vi "6700C Wrapper.vi"(6 "Measurement Type":i32(ring)=1 items=["Current", "Voltage", "Power"], 7 "States":T2, 8 "error in":errorcluster, 9 "Enable Output":bool, 10 "Setting":T1={"Max Volt"=10.0, "Voltage Set"=0.01, "Current Lim"=0.5, "Source Type"=enum."Current", "Current Set"=0.01, "Max Current"=10.0, "Voltage Lim"=0.5}, 11 "Alias":string="PS1") -> (0 "error out":errorcluster, 1 "Error Message":string, 2 "Error":i32, 3 "Measurement":dbl=nan)   [LabVIEW 2021]
doc: "This is a wrapper to support Keysight N6700C."
uses:
  Controls/PS States.ctl
  Load INI/Controls/PowerSupply_Data.ctl
  <instrlib>/Agilent N6700 Series/Agilent N6700 Series.lvlib
panel:
  # "This wrapper has only been tested with N6773A and\nN6744B PS Modules (loaded in N6700C mainframe\nall other models are disabled unless tested and added to list"
  # "Voltage Src"
  # "Current Src"
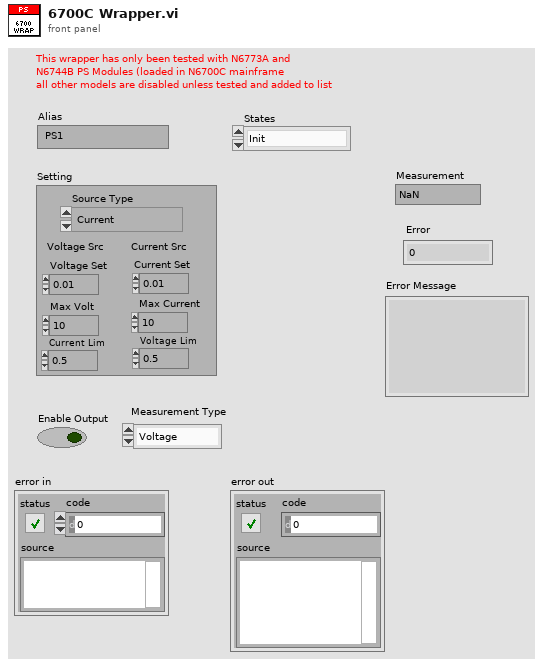
[diagram p1: front panel]
types:
  T1 = cluster{"Max Volt":dbl, "Voltage Set":dbl, "Current Lim":dbl, "Source Type":enum16{"Voltage", "Current"}, "Current Set":dbl, "Max Current":dbl, "Voltage Lim":dbl}
  T2 = typedef "PS States.ctl" = enum16{"Init", "Config", "Enable Output", "Measure", "Close"}
  T3 = cluster{"Channel Name":string, "VISA resource name":refnum<visa-resource-name>}
  T4 = typedef "PowerSupply_Data.ctl" = cluster{"Alias":string, "Device":string, "Channel name":string}
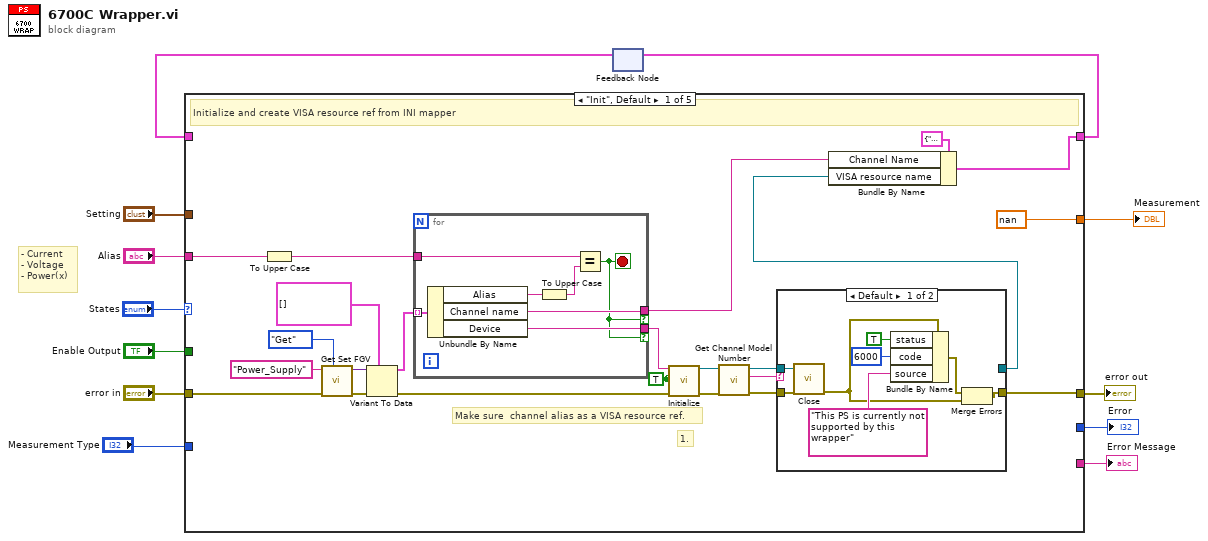
[diagram p0: block diagram]
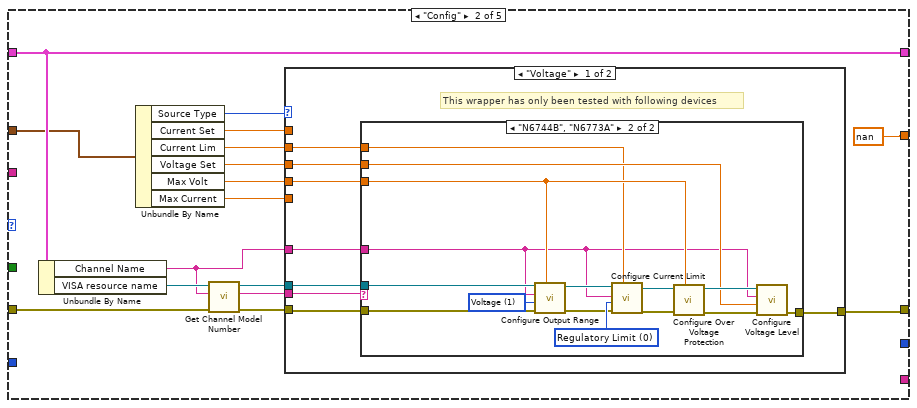
[diagram p3: hidden frame]
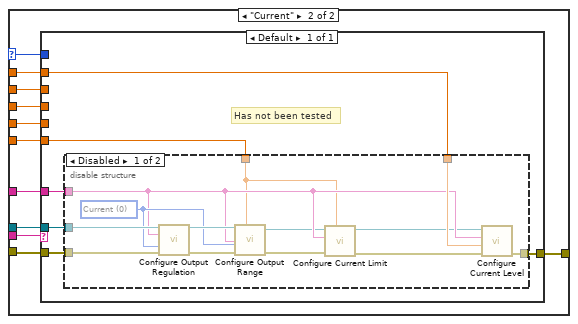
[diagram p5: hidden frame]
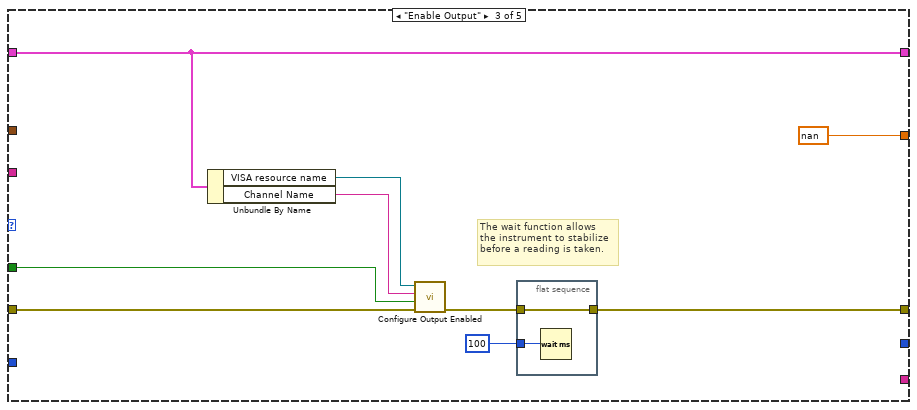
[diagram p7: hidden frame]
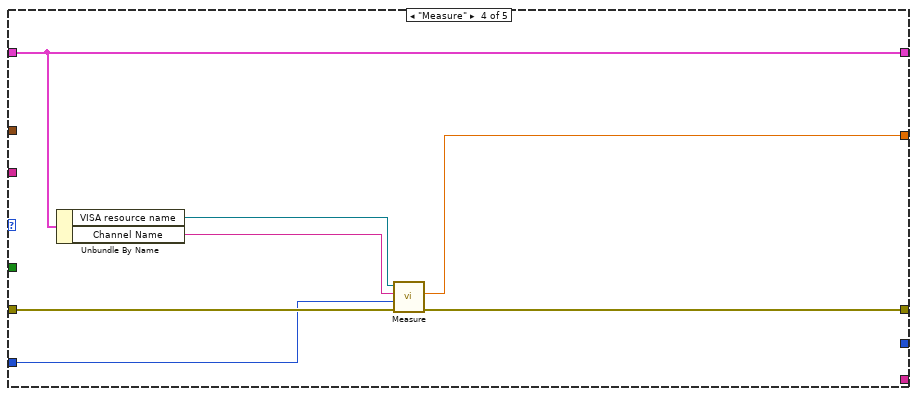
[diagram p8: hidden frame]
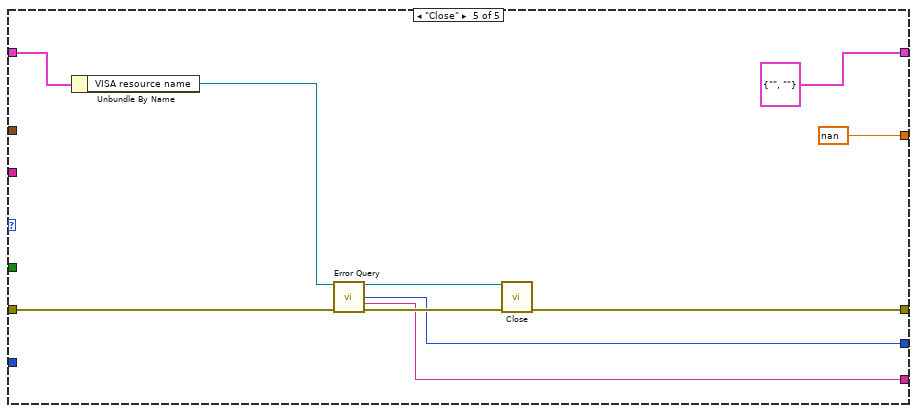
[diagram p9: hidden frame]
diagram:
  # "- Current\n- Voltage\n- Power(x)"
  n1 = feedback #1() -> (w8:T3)  [unwired: 1 in]
  n2 = case shown="\"Init\", Default" "States" {
    tunnel: "error in" -> [w33 w66 w132 w138 w148]
    tunnel: [w15 w61 w126 w140 w144] -> w10
    tunnel: [w34 w68 w131 w139 T3 {"Channel Name"="", "VISA resource name"=""}] -> w9
    tunnel: w8 -> [_ w68 w131 w139 w151]
    tunnel: [nan nan nan w141 nan] -> w4
    tunnel: "Enable Output" -> [_ _ w129 _ _]
    tunnel: "Setting" -> [_ w67 _ _ _]
    tunnel: "Alias" -> [w27 _ _ _ _]
    tunnel: [_ _ _ _ w143] -> w3
    tunnel: [_ _ _ _ w142] -> w2
    tunnel: "Measurement Type" -> [_ _ _ w135 _]
    frame "Init", Default {
      w23 = TRUE ("Reset? (T: Yes)")
      # "1."
      # "Make sure  channel alias as a VISA resource ref."
      # "Initialize and create VISA resource ref from INI mapper"
      n3 = To Upper Case(1:w27) -> (0:w26:string)
      n4 = call "Get Set FGV.vi"("Method (Get)"=enum16{"Get", "Set"}."Get", "error in"=w33, "Name"="Power_Supply") -> ("error out"=w31:errorcluster, "Data out"=w30:variant)  [unwired: 7 in]
      n5 = Variant To Data(error in=w31, type=T4[] [], Variant=w30) -> (data=w28:T4[], error out=w20:errorcluster)
      n6 = for {
        tunnel: w28 -> [w52] mode=indexing
        tunnel: w26 -> [w51]
        tunnel: [w48] -> w25 if=w46
        tunnel: [w47] -> w24 if=w46
        stop <- w46 stop-if-true
        n7 = Unbundle By Name(w52) -> ("Alias"=w49:string, "Channel name"=w47:string, "Device"=w48:string)
        n8 = To Upper Case(1:w49) -> (0:w50:string)
        n9 = Equal?(x=w51, y=w50) -> (x = y?=w46:bool)
      }
      n10 = call <instrlib>:"Initialize.vi"("VISA resource name"=w25, "ID Query? (T: Yes)"=w23, "Reset? (T: Yes)"=w23, "error in (no error)"=w20) -> ("VISA resource name out"=w18:refnum<visa-resource-name>, "error out"=w19:errorcluster)  [unwired: 10 in]
      n11 = call <instrlib>:"Get Channel Model Number.vi"("error in (no error)"=w19, "VISA resource name"=w18) -> ("error out"=w16:errorcluster, "Model Number"=w17:string, "VISA resource name out"=w14:refnum<visa-resource-name>)  [unwired: 7 in]
      n12 = case shown="Default" w17 {
        tunnel: w16 -> [w43 w45]
        tunnel: [w37 w45] -> w15
        tunnel: w14 -> [w42 w44]
        tunnel: [_ w44] -> w13
        frame Default {
          n13 = call <instrlib>:"Close.vi"("VISA resource name"=w42, "error in (no error)"=w43) -> ("error out"=w36:errorcluster)  [unwired: 13 in]
          n14 = Bundle By Name(cluster=w36, "status"=TRUE, "code"=6000, "source"="This PS is currently not supported by this wrapper") -> (w38:errorcluster)
          n15 = Merge Errors(w38, w36) -> (w37:errorcluster)
        }
        frame "N6744B", "N6773A" {
        }
      }
      n16 = Bundle By Name(cluster=T3 {"Channel Name"="", "VISA resource name"=""}, "Channel Name"=w24, "VISA resource name"=w13) -> (w34:T3)
    }
    frame "Config" {
      n17 = Unbundle By Name(w68) -> ("Channel Name"=w53:string, "VISA resource name"=w64:refnum<visa-resource-name>)
      n18 = Unbundle By Name(w67) -> ("Source Type"=w55:enum16{"Voltage", "Current"}, "Current Set"=w56:dbl, "Current Lim"=w60:dbl, "Voltage Set"=w58:dbl, "Max Volt"=w59:dbl, "Max Current"=w54:dbl)
      n19 = call <instrlib>:"Get Channel Model Number.vi"("error in (no error)"=w66, "Channel Name (1)"=w53, "VISA resource name"=w64) -> ("error out"=w65:errorcluster, "Model Number"=w57:string, "VISA resource name out"=w63:refnum<visa-resource-name>)  [unwired: 6 in]
      n20 = case shown="\"Voltage\"" w55 {
        selector: w55 -> [_ w94]
        tunnel: w53 -> [w70 w98]
        tunnel: w65 -> [w71 w102]
        tunnel: w63 -> [w72 w103]
        tunnel: [w75 w97] -> w61
        tunnel: w60 -> [w73 w101]
        tunnel: w59 -> [w74 w100]
        tunnel: w58 -> [w76 w99]
        tunnel: w57 -> [w69 w96]
        tunnel: w56 -> [_ w95]
        tunnel: w54 -> [_ w93]
        frame "Voltage" {
          # "This wrapper has only been tested with following devices"
          n21 = case shown="\"N6744B\", \"N6773A\"" w69 {
            tunnel: w76 -> [_ w86]
            tunnel: [w77 w84] -> w75
            tunnel: w74 -> [_ w83]
            tunnel: w73 -> [_ w82]
            tunnel: w72 -> [_ w81]
            tunnel: w71 -> [w77 w80]
            tunnel: w70 -> [_ w79]
            frame Default {
            }
            frame "N6744B", "N6773A" {
              w78 = 1 items=["Voltage"=1, "Current"=0] ("Range Type (1: Voltage)")
              w92 = 0 items=["Regulatory Limit", "Trip Limit"] ("Behavior (0: Regulatory Limit)")
              n22 = call <instrlib>:"Configure Output Range.vi"("Range (0.0)"=w83, "error in (no error)"=w80, "Range Type (1: Voltage)"=w78, "Channel Name (1)"=w79, "VISA resource name"=w81) -> ("error out"=w90:errorcluster, "VISA resource name out"=w91:refnum<visa-resource-name>)  [unwired: 5 in]
              n23 = call <instrlib>:"Configure Current Limit.vi"("Limit (0.0 amps)"=w82, "error in (no error)"=w90, "Behavior (0: Regulatory Limit)"=w92, "Channel Name (1)"=w79, "VISA resource name"=w91) -> ("error out"=w89:errorcluster, "VISA resource name out"=w87:refnum<visa-resource-name>)  [unwired: 5 in]
              n24 = call <instrlib>:"Configure Over Voltage Protection.vi"("Limit (0.0 volts)"=w83, "error in (no error)"=w89, "VISA resource name"=w87) -> ("error out"=w85:errorcluster, "VISA resource name out"=w88:refnum<visa-resource-name>)  [unwired: 7 in]
              n25 = call <instrlib>:"Configure Voltage Level.vi"("error in (no error)"=w85, "Level  (0.0 volts)"=w86, "Channel Name (1)"=w79, "VISA resource name"=w88) -> ("error out"=w84:errorcluster)  [unwired: 6 in, 1 out]
            }
          }
        }
        frame "Current" {
          n26 = case shown="Default" w96 {
            tunnel: w103 -> [w109]
            tunnel: w102 -> [w108]
            tunnel: w101 -> [_]
            tunnel: w100 -> [_]
            tunnel: w99 -> [_]
            tunnel: w98 -> [w105]
            tunnel: [w107] -> w97
            tunnel: w95 -> [w106]
            tunnel: w94 -> [_]
            tunnel: w93 -> [w104]
            frame Default {
              # "Has not been tested"
              n27 = disable-structure shown="Disabled" {
                disable-tunnel: w109 -> [w122 _]
                disable-tunnel: w108 -> [w121 w123]
                disable-tunnel: [w117 w123] -> w107
                disable-tunnel: w106 -> [w116 _]
                disable-tunnel: w105 -> [w115 _]
                disable-tunnel: w104 -> [w110 _]
                frame Disabled {
                  w118 = 0 items=["Voltage"=1, "Current"=0] ("Output Regulation Priority (1: Voltage)")
                  n28 = call <instrlib>:"Configure Output Regulation.vi"("VISA resource name"=w122, "Channel Name (1)"=w115, "Output Regulation Priority (1: Voltage)"=w118, "error in (no error)"=w121) -> ("VISA resource name out"=w119:refnum<visa-resource-name>, "error out"=w120:errorcluster)  [unwired: 10 in]
                  n29 = call <instrlib>:"Configure Output Range.vi"("Range (0.0)"=w110, "error in (no error)"=w120, "Range Type (1: Voltage)"=w118, "Channel Name (1)"=w115, "VISA resource name"=w119) -> ("error out"=w112:errorcluster, "VISA resource name out"=w113:refnum<visa-resource-name>)  [unwired: 5 in]
                  n30 = call <instrlib>:"Configure Current Limit.vi"("Limit (0.0 amps)"=w110, "error in (no error)"=w112, "Channel Name (1)"=w115, "VISA resource name"=w113) -> ("error out"=w111:errorcluster, "VISA resource name out"=w114:refnum<visa-resource-name>)  [unwired: 6 in]
                  n31 = call <instrlib>:"Configure Current Level.vi"("error in (no error)"=w111, "Level  (0.0 amps)"=w116, "Channel Name (1)"=w115, "VISA resource name"=w114) -> ("error out"=w117:errorcluster)  [unwired: 6 in, 1 out]
                }
                frame Enabled {
                }
              }
            }
          }
        }
      }
    }
    frame "Enable Output" {
      # "The wait function allows \nthe instrument to stabilize\nbefore a reading is taken."
      n32 = Unbundle By Name(w131) -> ("VISA resource name"=w128:refnum<visa-resource-name>, "Channel Name"=w130:string)
      n33 = call <instrlib>:"Configure Output Enabled.vi"("error in (no error)"=w132, "Enable Output (False)"=w129, "Channel Name (1)"=w130, "VISA resource name"=w128) -> ("error out"=w127:errorcluster)  [unwired: 6 in, 1 out]
      n34 = flat-sequence {
        tunnel: [w134] -> w126
        tunnel: w127 -> [w134]
        tunnel: u32 100 ("milliseconds to wait") -> [w133]
        frame #0 {
          n35 = Wait (ms)(milliseconds to wait=w133) -> ()  [unwired: 1 out]
        }
      }
    }
    frame "Measure" {
      n36 = Unbundle By Name(w139) -> ("VISA resource name"=w137:refnum<visa-resource-name>, "Channel Name"=w136:string)
      n37 = call <instrlib>:"Measure.vi"("error in (no error)"=w138, "Measurement Type (1: Voltage)"=w135, "Channel Name (1)"=w136, "VISA resource name"=w137) -> ("error out"=w140:errorcluster, "Measurement"=w141:dbl)  [unwired: 5 in, 1 out]
    }
    frame "Close" {
      n38 = Unbundle By Name(w151) -> ("VISA resource name"=w146:refnum<visa-resource-name>)
      n39 = call <instrlib>:"Error Query.vi"("VISA resource name"=w146, "error in (no error)"=w148) -> ("VISA resource name out"=w145:refnum<visa-resource-name>, "Error"=w143:i32, "Error Message"=w142:string, "error out"=w147:errorcluster)  [unwired: 10 in]
      n40 = call <instrlib>:"Close.vi"("VISA resource name"=w145, "error in (no error)"=w147) -> ("error out"=w144:errorcluster)  [unwired: 13 in]
    }
  }
  "error out" <- w10
  "Measurement" <- w4
  "Error" <- w3
  "Error Message" <- w2
  n41 = feedback-in #1(w9) -> ()
